vi "FPGA main.vi"() -> ()   [LabVIEW 2020]
uses:
  <vilib>/Platform/TimedLoop/XDataNode/timing_clust.ctl
  <vilib>/Platform/TimedLoop/XDataNode/nitl_modes.ctl
  <vilib>/Platform/TimedLoop/XDataNode/wakeup.ctl
  <vilib>/rvi/Emulation/niFpgaSctlEmulationGetInTimedLoop.vi
  <vilib>/rvi/Emulation/niFpgaEmulationReportErrorSimple.vi
  <vilib>/rvi/Emulation/niFpgaGetClockAttributes.vi
  <vilib>/rvi/Emulation/niFpgaCriticalErrorInLSC.vi
  <vilib>/rvi/eio/common/nirviEmuTemplateMethod_errors.vi
  <vilib>/rvi/interface/RandomDataEmulation/niFpgaRandomDataHandleErrors.vi
  <vilib>/Platform/TimedLoop/XDataNode/XDataNode.xnode
  <vilib>/eio/EIONode/EIONode.xnode
  <vilib>/rvi/DataTransferAndStorage/Container/XNode/niFpgaContainer.xnode
  <vilib>/rvi/interface/RandomDataEmulation/nirviRandomDataFpgaReadWriteTemplate.vi
  <vilib>/Platform/TimedLoop/XDataNode/XDNodeRunTimeDep.lvlib
panel:
  out "Cumulative timeout 2":bool
  out "Instant timeout 2":bool
  in  "Delay DAQ loop by n ticks":u32
  out "Instant timeout":bool
  out "Cumulative timeout":bool
  out "loop time":u32
  in  "stop":bool
  out "Init Done":bool
  in  "Start Acquisition":bool
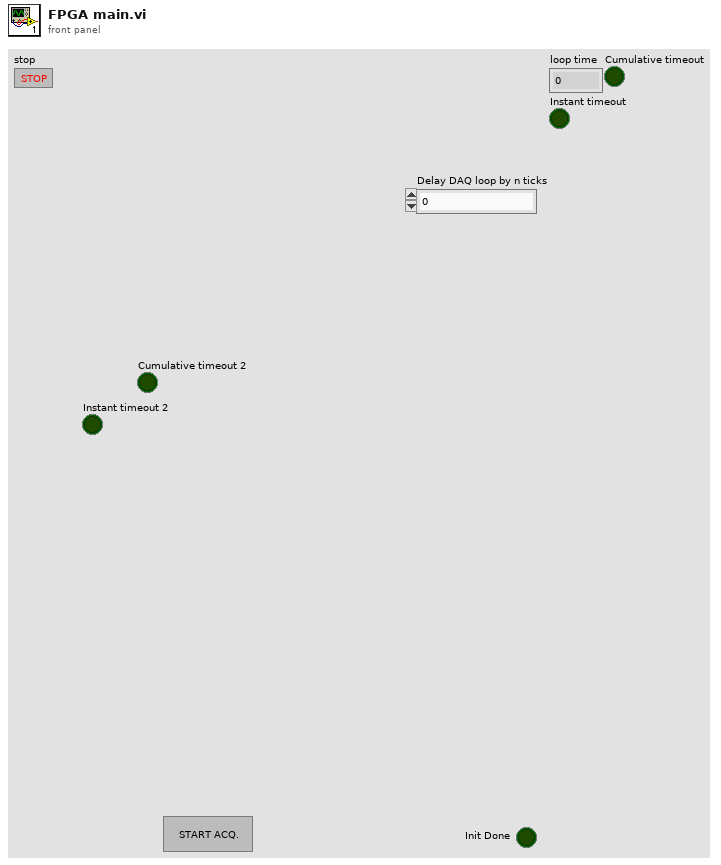
[diagram p1: front panel]
types:
  T1 = typedef "XDNodeRunTimeDep.lvlib/timing_clust.ctl" = cluster{"Expected End [f-1]":u64, "Actual End [f-1]":u64, "Finished Late? [f-1]":bool, "Expected End [i-1]":u64, "Actual End [i-1]":u64, "Finished Late? [i-1]":bool, "Expected Start [i]":u64, "Actual Start [i]":u64, "Expected Start [f]":u64, "Actual Start [f]":u64, "Source Name":string, "Structure Name":string, "Period":i64, "Deadline":i64, "Offset":i64, "Start":i64, "Priority":i32, "Timeout":i32, "Mode":T2, "Wakeup Reason":T3, "Error":errorcluster, "Source Type":string, "Secondary Source Type":string, "Global End Time":u64, "Global Start Time":u64, "Frame Duration":u64, "Iteration Duration":u64, "Assigned CPU":i32, "I/O Scan Engine Mode":u32}
  T2 = typedef "XDNodeRunTimeDep.lvlib/nitl_modes.ctl" = enum32{"No Change", "Process missed periods, maintain original phase", "Discard missed periods, maintain original phase", "Process missed periods, ignore original phase", "Discard missed periods, ignore original phase"}
  T3 = typedef "XDNodeRunTimeDep.lvlib/wakeup.ctl" = enum32{"Normal", "Aborted", "Asynchronous wakeup", "Timing source error", "Timed loop error", "Timeout"}
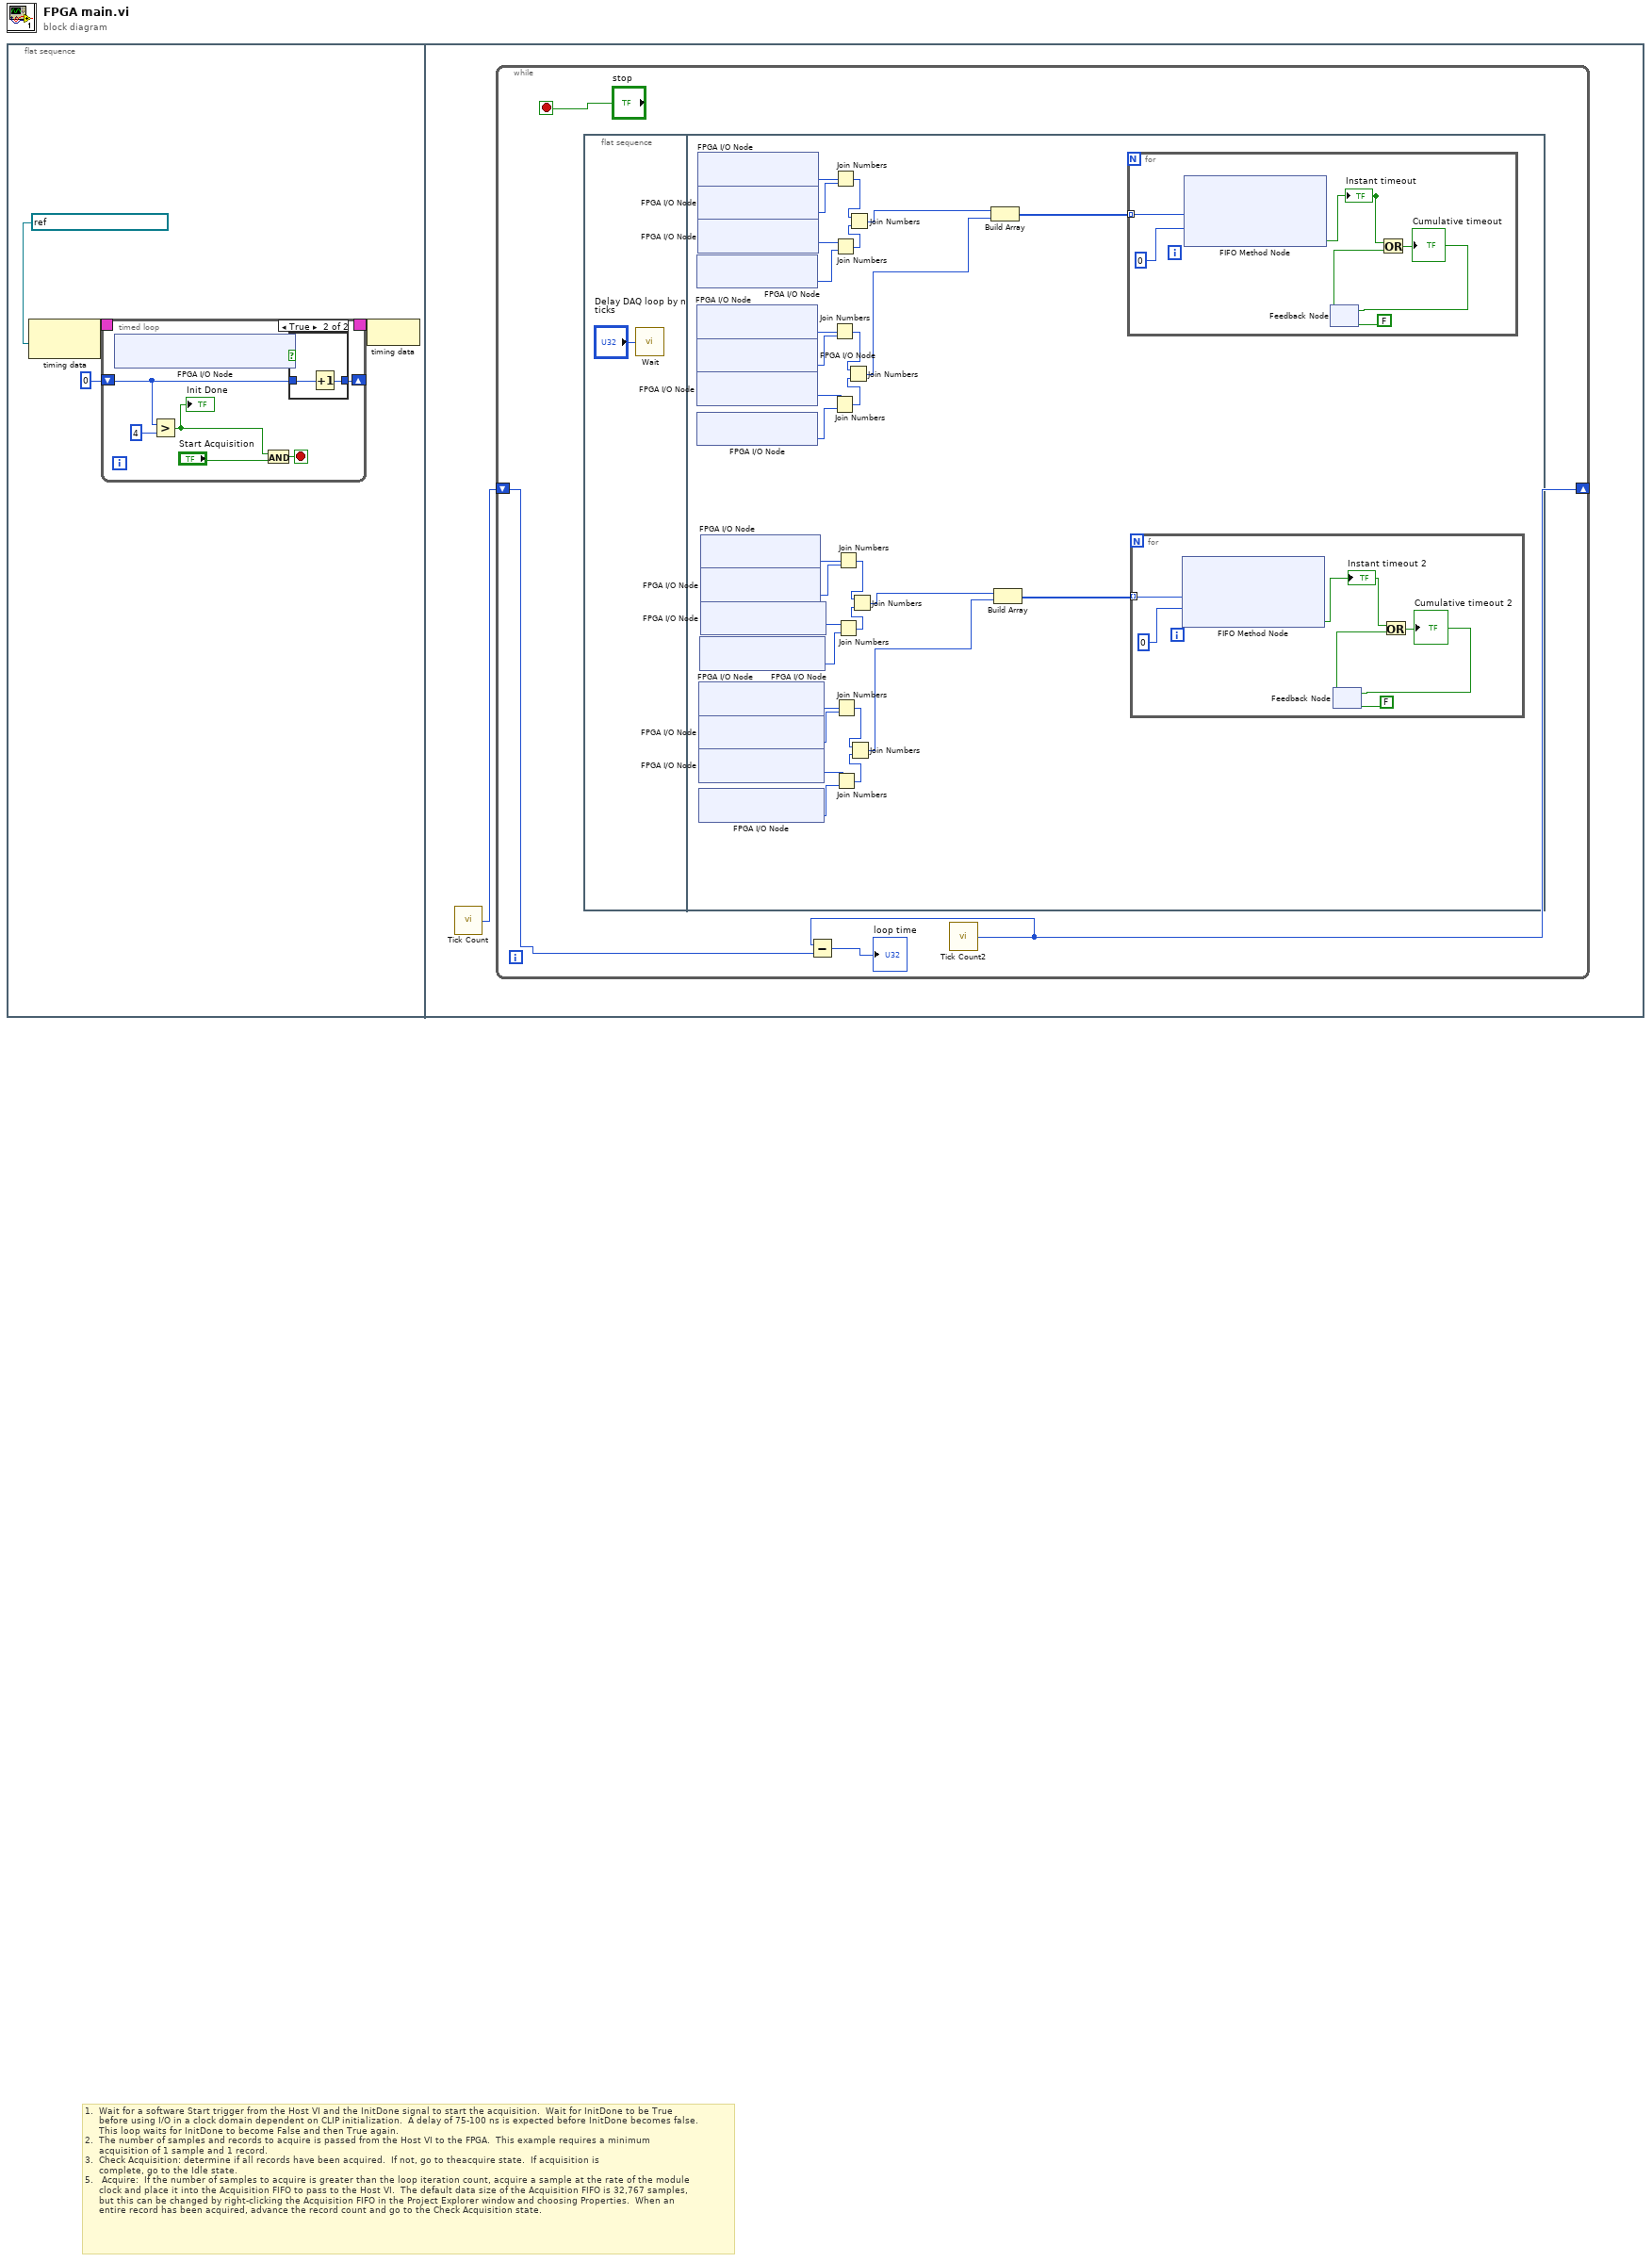
[diagram p0: block diagram]
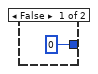
[diagram p2: hidden frame]
diagram:
  # "1.  Wait for a software Start trigger from the Host VI and the InitDone signal to start the acquisition.  Wait for InitDone to be True \n     before using I/O in a clock domain dependent on CLIP initialization.  A delay of 75-100 ns is expected before InitDone becomes false.  \n     This loop waits for InitDone to become False and then True again.\n2.  The number of samples and records to acquire is passed from the Host VI to the FPGA.  This example requires a minimum \n     acquisition of 1 sample and 1 record.\n3.  Check Acquisition: determine if all records have been acquired.  If not, go to theacquire state.  If acquisition is \n     complete, go to the Idle state.  \n5.   Acquire:  If the number of samples to acquire is greater than the loop iteration count, acquire a sample at the rate of the module \n     clock and place it into the Acquisition FIFO to pass to the Host VI.  The default data size of the Acquisition FIFO is 32,767 samples, \n     but this can be changed by right-clicking the Acquisition FIFO in the Project Explorer window and choosing Properties.  When an \n     entire record has been acquired, advance the record count and go to the Check Acquisition state."
  n1 = flat-sequence {
    frame #0 {
      n2 = node-c288(refnum<k21> "40 MHz Onboard Clock" ("Source Name")) -> (w4:T1)
      n3 = timed-loop {
        shift-right: [w10] -> _
        shift-left: u16 0 -> [w9]
        timing: w4 -> [_]
        timing-out: [_] -> w3
        stop <- w7 stop-if-true
        n4 = xnode "FPGA I/O Node"() -> ("IO Module\\Initialization Done"=w11:bool)  [unwired: 1 in, 1 out]
        n5 = Greater?(x=w9, y=u16 4) -> (0:w5:bool)
        "Init Done" <- w5
        n6 = And(x=w5, y="Start Acquisition") -> (x .and. y?=w7:bool)
        n7 = case shown="True" w11 {
          tunnel: [u16 0 w14] -> w10
          tunnel: w9 -> [_ w13]
          frame False {
          }
          frame True {
            n8 = Increment(x=w13) -> (x+1=w14:u16)
          }
        }
      }
      n9 = node-c288(w3) -> ()
    }
    frame #1 {
      n10 = call "Tick Count"() -> ("Tick Count(Ticks)"=w21:u32)
      n11 = while {
        shift-right: [w22] -> _
        shift-left: w21 -> [w23]
        stop <- "stop" stop-if-true
        n12 = flat-sequence {
          frame #0 {
            n13 = call "Wait"("Count(Ticks)"="Delay DAQ loop by n ticks") -> ()  [unwired: 1 out]
          }
          frame #1 {
            n14 = xnode "FPGA I/O Node"() -> ("IO Module\\AI A3"=w52:i16)  [unwired: 1 in, 1 out]
            n15 = xnode "FPGA I/O Node"() -> ("IO Module\\AI A4"=w49:i16)  [unwired: 1 in, 1 out]
            n16 = xnode "FPGA I/O Node"() -> ("IO Module\\AI A5"=w50:i16)  [unwired: 1 in, 1 out]
            n17 = xnode "FPGA I/O Node"() -> ("IO Module\\AI A6"=w51:i16)  [unwired: 1 in, 1 out]
            n18 = xnode "FPGA I/O Node"() -> ("IO Module\\AI A7"=w46:i16)  [unwired: 1 in, 1 out]
            n19 = xnode "FPGA I/O Node"() -> ("IO Module\\AI A0"=w45:i16)  [unwired: 1 in, 1 out]
            n20 = xnode "FPGA I/O Node"() -> ("IO Module\\AI A1"=w55:i16)  [unwired: 1 in, 1 out]
            n21 = xnode "FPGA I/O Node"() -> ("IO Module\\AI A2"=w56:i16)  [unwired: 1 in, 1 out]
            n22 = xnode "FPGA I/O Node"() -> ("IO Module\\AI B12"=w34:i16)  [unwired: 1 in, 1 out]
            n23 = xnode "FPGA I/O Node"() -> ("IO Module\\AI B13"=w35:i16)  [unwired: 1 in, 1 out]
            n24 = xnode "FPGA I/O Node"() -> ("IO Module\\AI B14"=w36:i16)  [unwired: 1 in, 1 out]
            n25 = xnode "FPGA I/O Node"() -> ("IO Module\\AI B15"=w31:i16)  [unwired: 1 in, 1 out]
            n26 = xnode "FPGA I/O Node"() -> ("IO Module\\AI B11"=w37:i16)  [unwired: 1 in, 1 out]
            n27 = xnode "FPGA I/O Node"() -> ("IO Module\\AI B8"=w30:i16)  [unwired: 1 in, 1 out]
            n28 = xnode "FPGA I/O Node"() -> ("IO Module\\AI B9"=w40:i16)  [unwired: 1 in, 1 out]
            n29 = xnode "FPGA I/O Node"() -> ("IO Module\\AI B10"=w41:i16)  [unwired: 1 in, 1 out]
            n30 = Join Numbers(hi=w49, lo=w50) -> ((hi.lo)=w48:u32)
            n31 = Join Numbers(hi=w51, lo=w46) -> ((hi.lo)=w47:u32)
            n32 = Join Numbers(hi=w45, lo=w55) -> ((hi.lo)=w54:u32)
            n33 = Join Numbers(hi=w56, lo=w52) -> ((hi.lo)=w53:u32)
            n34 = Join Numbers(hi=w34, lo=w35) -> ((hi.lo)=w33:u32)
            n35 = Join Numbers(hi=w36, lo=w31) -> ((hi.lo)=w32:u32)
            n36 = Join Numbers(hi=w30, lo=w40) -> ((hi.lo)=w39:u32)
            n37 = Join Numbers(hi=w41, lo=w37) -> ((hi.lo)=w38:u32)
            n38 = Join Numbers(hi=w48, lo=w47) -> ((hi.lo)=w44:u64)
            n39 = Join Numbers(hi=w54, lo=w53) -> ((hi.lo)=w43:u64)
            n40 = Join Numbers(hi=w33, lo=w32) -> ((hi.lo)=w29:u64)
            n41 = Join Numbers(hi=w39, lo=w38) -> ((hi.lo)=w28:u64)
            n42 = Build Array(w43, w44) -> (w42:u64[])
            n43 = Build Array(w28, w29) -> (w27:u64[])
            n44 = for {
              tunnel: w42 -> [w67] mode=indexing
              n45 = xnode ("FIFO Method Node")("Element"=w67, "Timeout"=0) -> ("Timed Out?"=w63:bool)  [unwired: 1 in, 1 out]
              "Instant timeout" <- w63
              n46 = feedback #1(FALSE) -> (w65:bool)
              n47 = Or(x=w63, y=w65) -> (x .or. y?=w64:bool)
              "Cumulative timeout" <- w64
              n48 = feedback-in #1(w64) -> ()
            }
            n49 = for {
              tunnel: w27 -> [w59] mode=indexing
              n50 = xnode ("FIFO Method Node")("Element"=w59, "Timeout"=0) -> ("Timed Out?"=w57:bool)  [unwired: 1 in, 1 out]
              "Instant timeout 2" <- w57
              n51 = feedback #2(FALSE) -> (w61:bool)
              n52 = Or(x=w57, y=w61) -> (x .or. y?=w60:bool)
              "Cumulative timeout 2" <- w60
              n53 = feedback-in #2(w60) -> ()
            }
          }
        }
        n54 = call "Tick Count2"() -> ("Tick Count(Ticks)"=w22:u32)
        n55 = Subtract(x=w22, y=w23) -> (x-y=→"loop time":u32)
      }
    }
  }
